vi "Data Type to Test Executives.vi"(8 "error in (no error)":errorcluster, 11 "Data Type":refnum<class "Data Type.lvclass">) -> (0 "error out":errorcluster, 3 "Test Executive Refs":refnum<data-value>[](array[refnum]))   [LabVIEW 2017, in "Custom Type Test Executive.lvlib" / "Test Executive 1D.lvclass"]
uses:
  <vilib>/gpm_packages/@cs/test-executive/Source/Custom Type Test Executive/Test Executive 1D Data Type/Test Executive 1D.lvclass
  <vilib>/gpm_packages/@cs/data-type-serializer/source/Data Type/Data Type.lvclass
  <vilib>/gpm_packages/@cs/test-executive/Source/Test Executive/ITestExecutive/ITest Executive.lvclass
  <vilib>/gpm_packages/@cs/test-executive/Source/Custom Type Test Executive/Test Executive 1D Data Type/Test Executive 1D.lvclass/Test Executive 1D.ctl
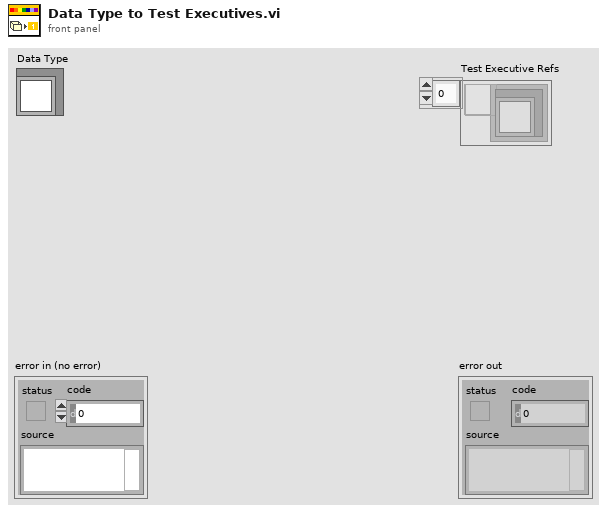
[diagram p1: front panel]
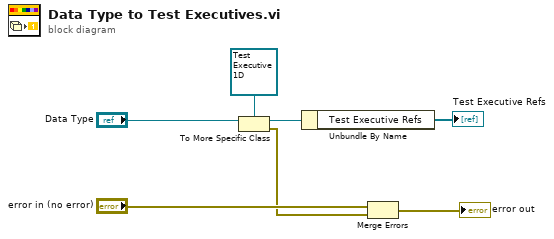
[diagram p0: block diagram]
diagram:
  n1 = To More Specific Class(target class=refnum<class "Test Executive 1D.lvclass"> refnum ("Boolean out"), reference="Data Type") -> (specific class reference=w4:refnum<class "Test Executive 1D.lvclass">, error out=w2:errorcluster)  [unwired: 1 in]
  n2 = Unbundle By Name(w4) -> ("Test Executive Refs"=→"Test Executive Refs":refnum<data-value>[])
  n3 = Merge Errors("error in (no error)", w2) -> (→"error out":errorcluster)
